vi "DisableEnable_mono.vi"(0 "Control in":refnum<vi>, 9 "Action in":T1, 11 "error in (no error)":errorcluster) -> (15 "error out":errorcluster)   [LabVIEW 2012]
uses:
  type def/Hyde&Show.ctl
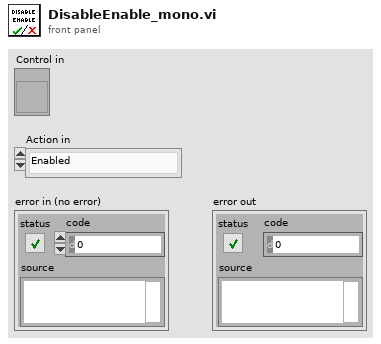
[diagram p1: front panel]
types:
  T1 = typedef "Hyde&Show.ctl" = enum8{"Enabled", "Disabled", " Grayed Out", "Hide"}
  T2 = enum8{"Enabled", "Disabled", "Disabled and Grayed Out"}
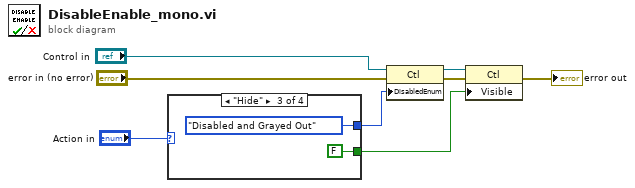
[diagram p0: block diagram]
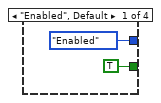
[diagram p2: hidden frame]
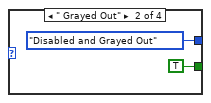
[diagram p3: hidden frame]
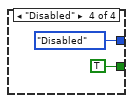
[diagram p4: hidden frame]
diagram:
  n1 = case shown="\"Hide\"" "Action in" {
    tunnel: [TRUE TRUE FALSE TRUE] -> w6
    tunnel: [T2."Enabled" ("Action") T2."Disabled and Grayed Out" ("Action") T2."Disabled and Grayed Out" ("Action") T2."Disabled" ("Action")] -> w7
    frame "Enabled", Default {
    }
    frame " Grayed Out" {
    }
    frame "Hide" {
    }
    frame "Disabled" {
    }
  }
  n2 = property class="Ctl"(reference="Control in", error in="error in (no error)", "DisabledEnum"=w7) -> (reference out=w1:refnum<vi>, error out=w2:errorcluster)
  n3 = property class="Ctl"(reference=w1, error in=w2, "Visible"=w6) -> (error out=→"error out":errorcluster)  [unwired: 1 out]
